vi "Periodic Tasks.vi"(8 "error in":errorcluster) -> ()   [LabVIEW 2016]
doc: "This VI runs in parallel to other tasks. It can contain as many user-defined periodic loops as you need. These can carry out PID or other sorts of timed response."
uses:
  <vilib>/Rock Robotics/WPI/Utilities/WPI_GetSetVariantRefNum.vi
  <vilib>/Rock Robotics/Network Tables/NT Read Number.vi
  <vilib>/Rock Robotics/Network Tables/NT Write Number.vi
  <vilib>/Rock Robotics/Network Tables/NT Read Boolean.vi
panel:
  out "Compressor Running":bool
  out "Compressor Monitoring":bool
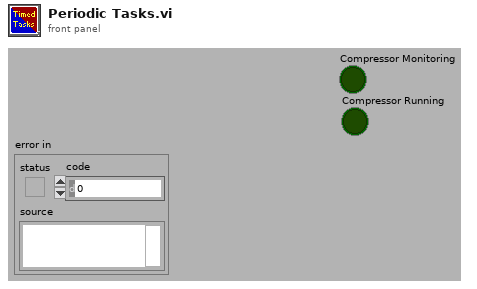
[diagram p1: front panel]
types:
  T1 = typedef "WPI_JoystickDevRef.ctl" = cluster{"Device":T2}
  T2 = typedef "WPI_JoystickDeviceEnum.ctl" = enum16{"USB 0", "USB 1", "USB 2", "USB 3", "USB 4", "USB 5"}
  T3 = cluster{"Buttons[0]":bool, "Buttons[1]":bool, "Buttons[2]":bool, "Buttons[3]":bool, "Buttons[4]":bool, "Buttons[5]":bool, "Buttons[6]":bool, "Buttons[7]":bool, "Buttons[8]":bool}
  T4 = typedef "WPI_AnalogChannelDevRef.ctl" = cluster{"DevStatus":errorcluster, "Analog Channel":T5}
  T5 = typedef "FPGA_AIChannel.ctl" = enum8{"AI 0", "AI 1", "AI 2", "AI 3", "AI MXP 0", "AI MXP 1", "AI MXP 2", "AI MXP 3", "Invalid"}
  T6 = typedef "WPI_RobotDriveDevRef.ctl" = cluster{"DevStatus":errorcluster, "Motors[]":T7[], "Square Inputs":bool, "Max Output":dbl}
  T7 = typedef "WPI_MotorControlDeviceRef.ctl" = cluster{"DeviceStatus":errorcluster, "Type":T8, "PWM":cluster{"PWM Channel":T9, "DeadBand":T10}, "CAN":cluster{"Device Number":u8, "SetOutput VI Ref":variant, "GetOutput VI Ref":variant, "Enable VI Ref":variant, "Disable VI Ref":variant, "Data":variant}, "Invert":bool}
  T8 = typedef "WPI_MotorControlType.ctl" = enum16{"PWM", "CAN"}
  T9 = typedef "FPGA_DIOPWMChannel.ctl" = enum8{"PWM 0", "PWM 1", "PWM 2", "PWM 3", "PWM 4", "PWM 5", "PWM 6", "PWM 7", "PWM 8", "PWM 9", "PWM MXP 0", "PWM MXP 1", "PWM MXP 2", "PWM MXP 3", "PWM MXP 4", "PWM MXP 5", "PWM MXP 6", "PWM MXP 7", "PWM MXP 8", "PWM MXP 9", "Invalid"}
  T10 = typedef "WPI_PWMDeadband.ctl" = cluster{"Name":string, "maxPositivePwm":i32, "minPositivePwm":i32, "centerPwm":i32, "maxNegativePwm":i32, "minNegativePwm":i32, "angularRange":u16}
  T11 = cluster{"JoystickDevRef":T1, "RobotDriveDevRef":T6, "JoystickDevRef":T1}
  T12 = typedef "WPI_CompressorDevRef.ctl" = cluster{"DevStatus":errorcluster, "Pneumatics Control Module":u8}
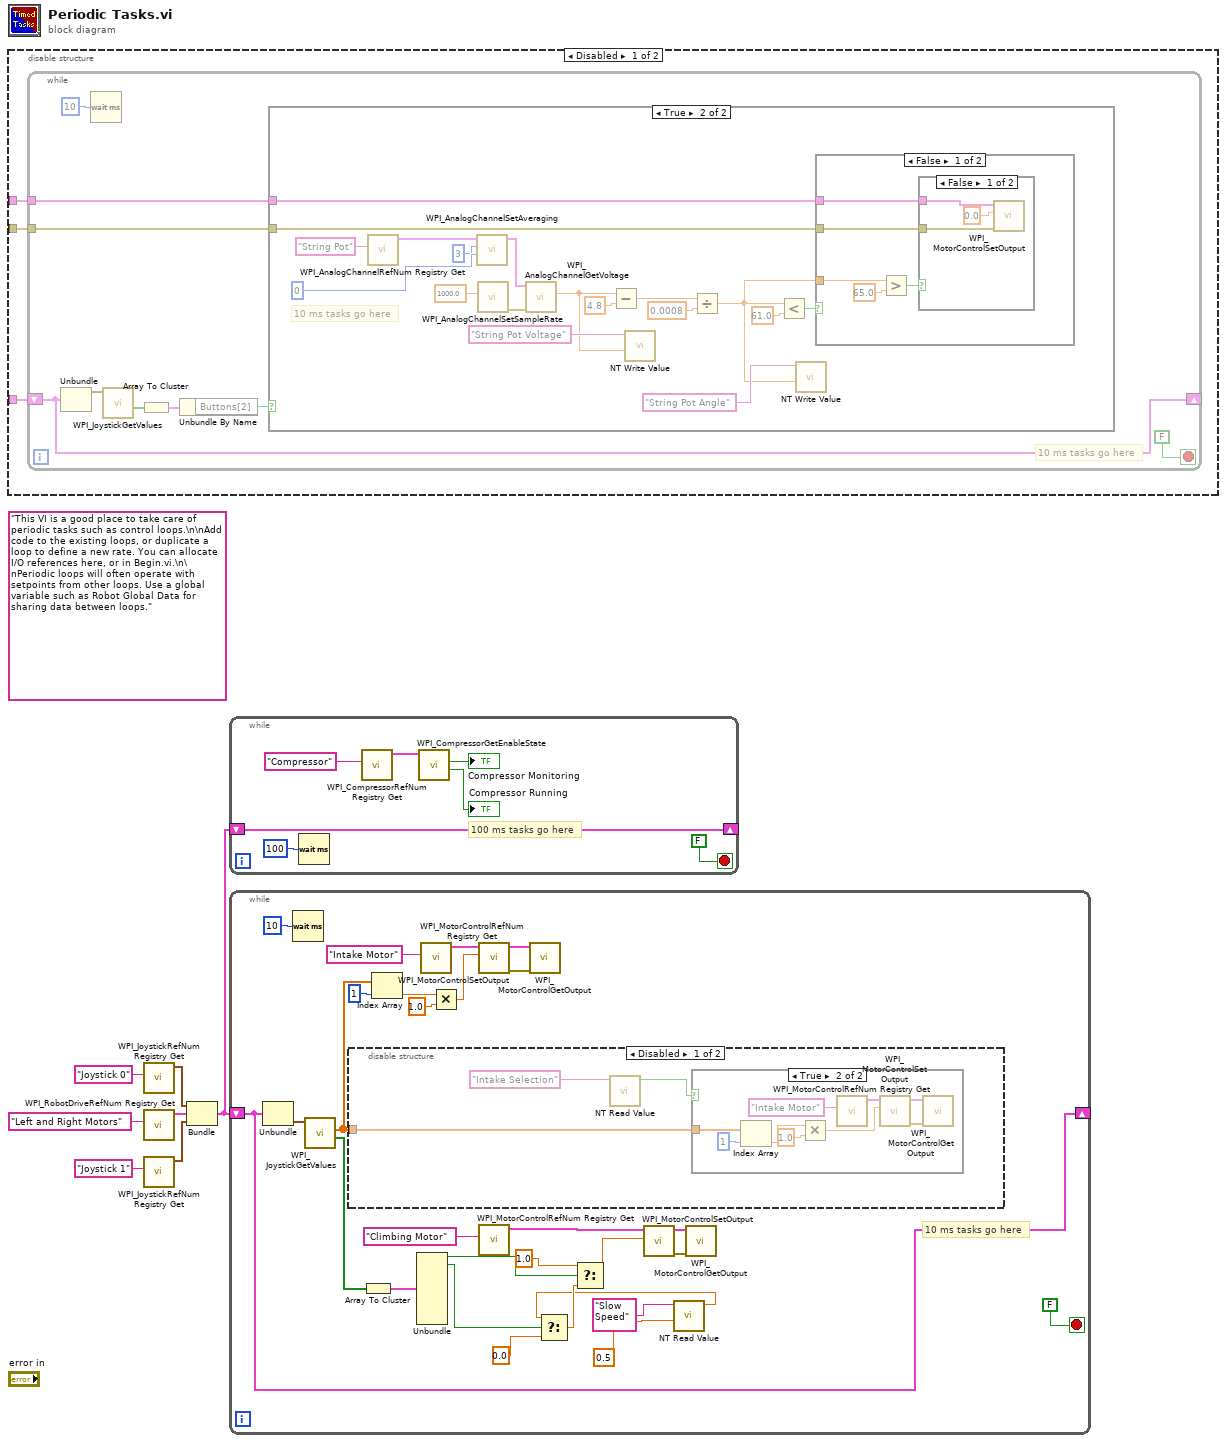
[diagram p0: block diagram]
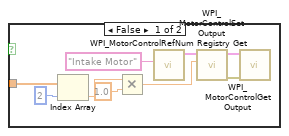
[diagram p2: hidden frame]
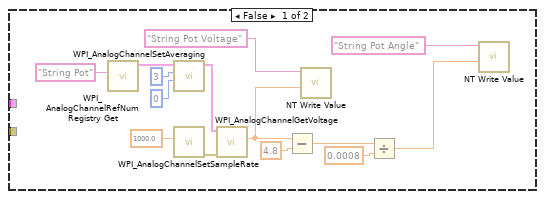
[diagram p4: hidden frame]
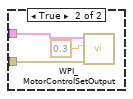
[diagram p5: hidden frame]
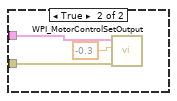
[diagram p6: hidden frame]
diagram:
  (unwired) "This VI is a good place to take care of periodic tasks such as control loops.\n\nAdd code to the existing loops, or duplicate a loop to define a new rate. You can allocate I/O references here, or in Begin.vi.\n\nPeriodic loops will often operate with setpoints from other loops. Use a global variable such as Robot Global Data for sharing data between loops."
  n1 = disable-structure shown="Disabled" {
    disable-tunnel: _ -> [w10 _]
    disable-tunnel: _ -> [w9 _]
    disable-tunnel: _ -> [w8 _]
    frame Disabled {
      n2 = while {
        shift-right: [w17] -> _
        shift-left: w8 -> [w17]
        tunnel: w10 -> [w12]
        tunnel: w9 -> [w11]
        stop <- FALSE stop-if-true
        # "10 ms tasks go here"
        n3 = Unbundle(w17) -> ("JoystickDevRef"=w16:T1)  [unwired: 2 out]
        n4 = Wait (ms)(milliseconds to wait=u32 10) -> ()  [unwired: 1 out]
        n5 = call <vilib>:"WPI_JoystickGetValues.vi"("JoystickDevRef"=w16) -> ("Buttons"=w15:bool[])  [unwired: 6 in, 4 out]
        n6 = Array To Cluster(array=w15) -> (cluster=w14:T3)
        n7 = Unbundle By Name(w14) -> ("Buttons[2]"=w13:bool)
        n8 = case shown="True" w13 {
          tunnel: w12 -> [_ w34]
          tunnel: w11 -> [_ w35]
          frame False {
            n9 = call <vilib>:"WPI_AnalogChannelRefNum Registry Get.vi"("refnum name"="String Pot") -> ("AIDeviceRef"=w24:T4)  [unwired: 9 in, 1 out]
            n10 = call <vilib>:"WPI_AnalogChannelSetAveraging.vi"("OversampleBits"=u8 0, "AverageBits"=u8 3 ("Average Bits"), "AIDeviceRef"=w24) -> ("AIDeviceRef"=w23:T4)  [unwired: 1 in, 7 out]
            n11 = call <vilib>:"WPI_AnalogChannelSetSampleRate.vi"("Samples Per Second (per channel)"=1000.0) -> ("error out"=w20:errorcluster)  [unwired: 4 in, 6 out]
            n12 = call <vilib>:"WPI_AnalogChannelGetVoltage.vi"("error in (no error)"=w20, "AIDeviceRef"=w23) -> ("Voltage"=w21:dbl)  [unwired: 9 out]
            n13 = Subtract(x=w21, y=4.8) -> (x-y=w30:dbl)
            n14 = call-poly <vilib>:"NT Write Value.vi"("Numeric"=w21, "Name"="String Pot Voltage") -> ()  [unwired: 9 in, 1 out]
            n15 = Divide(x=w30, y=0.0008) -> (x/y=w33:dbl)
            n16 = call-poly <vilib>:"NT Write Value.vi"("Numeric"=w33, "Name"="String Pot Angle") -> ()  [unwired: 9 in, 1 out]
          }
          frame True {
            # "10 ms tasks go here"
            n17 = call <vilib>:"WPI_AnalogChannelRefNum Registry Get.vi"("refnum name"="String Pot") -> ("AIDeviceRef"=w45:T4)  [unwired: 9 in, 1 out]
            n18 = call <vilib>:"WPI_AnalogChannelSetAveraging.vi"("OversampleBits"=u8 0, "AverageBits"=u8 3 ("Average Bits"), "AIDeviceRef"=w45) -> ("AIDeviceRef"=w46:T4)  [unwired: 1 in, 7 out]
            n19 = call <vilib>:"WPI_AnalogChannelSetSampleRate.vi"("Samples Per Second (per channel)"=1000.0) -> ("error out"=w40:errorcluster)  [unwired: 4 in, 6 out]
            n20 = call <vilib>:"WPI_AnalogChannelGetVoltage.vi"("error in (no error)"=w40, "AIDeviceRef"=w46) -> ("Voltage"=w39:dbl)  [unwired: 9 out]
            n21 = Subtract(x=w39, y=4.8) -> (x-y=w49:dbl)
            n22 = call-poly <vilib>:"NT Write Value.vi"("Numeric"=w39, "Name"="String Pot Voltage") -> ()  [unwired: 9 in, 1 out]
            n23 = Divide(x=w49, y=0.0008) -> (x/y=w37:dbl)
            n24 = Less?(x=w37, y=61.0) -> (x < y?=w36:bool)
            n25 = call-poly <vilib>:"NT Write Value.vi"("Numeric"=w37, "Name"="String Pot Angle") -> ()  [unwired: 9 in, 1 out]
            n26 = case shown="False" w36 {
              tunnel: w37 -> [w54 _]
              tunnel: w34 -> [w53 w64]
              tunnel: w35 -> [w52 w63]
              frame False {
                n27 = Greater?(x=w54, y=65.0) -> (0:w55:bool)
                n28 = case shown="False" w55 {
                  tunnel: w53 -> [w59 w62]
                  tunnel: w52 -> [w57 w61]
                  frame False {
                    n29 = call <vilib>:"WPI_MotorControlSetOutput.vi"("error in (no error)"=w57, "Output"=0.0, "MotorControlDevRef"=w59) -> ()  [unwired: 6 in, 3 out]
                  }
                  frame True {
                    n30 = call <vilib>:"WPI_MotorControlSetOutput.vi"("error in (no error)"=w61, "Output"=0.3, "MotorControlDevRef"=w62) -> ()  [unwired: 6 in, 3 out]
                  }
                }
              }
              frame True {
                n31 = call <vilib>:"WPI_MotorControlSetOutput.vi"("error in (no error)"=w63, "Output"=-0.3, "MotorControlDevRef"=w64) -> ()  [unwired: 6 in, 3 out]
              }
            }
          }
        }
      }
    }
    frame Enabled {
    }
  }
  n32 = call <vilib>:"WPI_JoystickRefNum Registry Get.vi"("refnum name"="Joystick 0") -> ("JoystickDevRef"=w5:T1)  [unwired: 1 in, 9 out]
  n33 = call <vilib>:"WPI_RobotDriveRefNum Registry Get.vi"("refnum name"="Left and Right Motors") -> ("RobotDriveDevRef"=w4:T6)  [unwired: 1 in, 9 out]
  n34 = call <vilib>:"WPI_JoystickRefNum Registry Get.vi"("refnum name"="Joystick 1") -> ("JoystickDevRef"=w2:T1)  [unwired: 1 in, 9 out]
  n35 = Bundle("JoystickDevRef"=w5, "RobotDriveDevRef"=w4, "JoystickDevRef"=w2) -> (w1:T11)  [unwired: 1 out]
  n36 = while {
    shift-right: [w70] -> _
    shift-left: w1 -> [w70]
    stop <- FALSE stop-if-true
    # "100 ms tasks go here"
    n37 = Wait (ms)(milliseconds to wait=u32 100) -> ()  [unwired: 1 out]
    n38 = call <vilib>:"WPI_CompressorRefNum Registry Get.vi"("refnum name"="Compressor") -> ("CompressorDevRef"=w68:T12)  [unwired: 9 in, 1 out]
    n39 = call <vilib>:"WPI_CompressorGetEnableState.vi"("CompressorDevRef"=w68) -> ("Compressor Running"=→"Compressor Running":bool, "Enabled"=→"Compressor Monitoring":bool)  [unwired: 7 in, 2 out]
  }
  n40 = while {
    shift-right: [w98] -> _
    shift-left: w1 -> [w98]
    stop <- FALSE stop-if-true
    # "10 ms tasks go here"
    n41 = Unbundle(w98) -> ("JoystickDevRef"=w97:T1)  [unwired: 2 out]
    n42 = Wait (ms)(milliseconds to wait=u32 10) -> ()  [unwired: 1 out]
    n43 = call <vilib>:"WPI_JoystickGetValues.vi"("JoystickDevRef"=w97) -> ("Buttons"=w96:bool[], "Axes"=w81:dbl[])  [unwired: 6 in, 3 out]
    n44 = disable-structure shown="Disabled" {
      disable-tunnel: w81 -> [w101 _]
      frame Disabled {
        n45 = call-poly <vilib>:"NT Read Value.vi"("Name"="Intake Selection" ("refnum name")) -> ("Boolean"=w102:bool)  [unwired: 9 in, 1 out]
        n46 = case shown="True" w102 {
          tunnel: w101 -> [w104 w113]
          frame False {
            n47 = Index Array(array=w104, index=2) -> (element=w107:dbl)
            n48 = Multiply(x=w107, y=1.0) -> (x*y=w108:dbl)
            n49 = call <vilib>:"WPI_MotorControlRefNum Registry Get.vi"("refnum name"="Intake Motor") -> ("MotorControlDevRef"=w105:T7)  [unwired: 9 in, 1 out]
            n50 = call <vilib>:"WPI_MotorControlSetOutput.vi"("Output"=w108, "MotorControlDevRef"=w105) -> ("error out"=w109:errorcluster, "MotorControlDevRef"=w106:T7)  [unwired: 7 in, 1 out]
            n51 = call <vilib>:"WPI_MotorControlGetOutput.vi"("error in"=w109, "MotorControlDevRef"=w106) -> ()  [unwired: 7 in, 3 out]
          }
          frame True {
            n52 = Index Array(array=w113, index=1) -> (element=w119:dbl)
            n53 = Multiply(x=w119, y=1.0) -> (x*y=w118:dbl)
            n54 = call <vilib>:"WPI_MotorControlRefNum Registry Get.vi"("refnum name"="Intake Motor") -> ("MotorControlDevRef"=w121:T7)  [unwired: 9 in, 1 out]
            n55 = call <vilib>:"WPI_MotorControlSetOutput.vi"("Output"=w118, "MotorControlDevRef"=w121) -> ("error out"=w117:errorcluster, "MotorControlDevRef"=w120:T7)  [unwired: 7 in, 1 out]
            n56 = call <vilib>:"WPI_MotorControlGetOutput.vi"("error in"=w117, "MotorControlDevRef"=w120) -> ()  [unwired: 7 in, 3 out]
          }
        }
      }
      frame Enabled {
      }
    }
    n57 = Array To Cluster(array=w96) -> (cluster=w92:T3)
    n58 = Index Array(array=w81, index=1) -> (element=w84:dbl)
    n59 = Unbundle(w92) -> ("Buttons[0]"=w91:bool, "Buttons[1]"=w79:bool)  [unwired: 7 out]
    n60 = call <vilib>:"WPI_MotorControlRefNum Registry Get.vi"("refnum name"="Intake Motor") -> ("MotorControlDevRef"=w82:T7)  [unwired: 9 in, 1 out]
    n61 = Multiply(x=w84, y=1.0) -> (x*y=w85:dbl)
    n62 = call <vilib>:"WPI_MotorControlSetOutput.vi"("Output"=w85, "MotorControlDevRef"=w82) -> ("error out"=w86:errorcluster, "MotorControlDevRef"=w83:T7)  [unwired: 7 in, 1 out]
    n63 = call <vilib>:"WPI_MotorControlRefNum Registry Get.vi"("refnum name"="Climbing Motor") -> ("MotorControlDevRef"=w95:T7)  [unwired: 9 in, 1 out]
    n64 = call <vilib>:"WPI_MotorControlGetOutput.vi"("error in"=w86, "MotorControlDevRef"=w83) -> ()  [unwired: 7 in, 3 out]
    n65 = call-poly <vilib>:"NT Read Value.vi"("Default Value"=0.5, "Name"="Slow Speed" ("refnum name")) -> ("Numeric"=w73:dbl)  [unwired: 8 in, 1 out]
    n66 = Select(t=w73, s=w79, f=0.0) -> (s? t:f=w76:dbl)
    n67 = Select(t=1.0, s=w91, f=w76) -> (s? t:f=w78:dbl)
    n68 = call <vilib>:"WPI_MotorControlSetOutput.vi"("Output"=w78, "MotorControlDevRef"=w95) -> ("error out"=w93:errorcluster, "MotorControlDevRef"=w94:T7)  [unwired: 7 in, 1 out]
    n69 = call <vilib>:"WPI_MotorControlGetOutput.vi"("error in"=w93, "MotorControlDevRef"=w94) -> ()  [unwired: 7 in, 3 out]
  }
